vi "Seq AE.vi"(0 "Action":enum16{"READ", "BUILD", "WRITE", "DELETE"}(ring), 3 "Cluster":T5 {"Laser Parameters Out"."STED Power (V)" scale=0.0..10.0; "Image Acquisition Parameters Out"."Z Steps Size (um)" min=0.0; "Image Acquisition Parameters Out"."Number of Z Steps" min=1; "Image Acquisition Parameters Out"."Frames Accumulations" min=1; "Image Acquisition Parameters Out"."Frames Per Capture" min=1; "Image Acquisition Parameters Out"."Line Accumulations" min=1; "Image Acquisition Parameters Out"."Image Format" items=["64 x 64"=64, "128 x 128"=128, "256 x 256"=256, "512 x 512"=512, "1024 x 1024"=1024, "2048 x 2048"=2048, "Customized..."=0]}) -> (9 "Array":T4(array[cluster]) {"Laser Parameters Out"."STED Power (V)" scale=0.0..10.0; "Image Acquisition Parameters Out"."Z Steps Size (um)" min=0.0; "Image Acquisition Parameters Out"."Number of Z Steps" min=1; "Image Acquisition Parameters Out"."Frames Accumulations" min=1; "Image Acquisition Parameters Out"."Frames Per Capture" min=1; "Image Acquisition Parameters Out"."Line Accumulations" min=1; "Image Acquisition Parameters Out"."Image Format" items=["64 x 64"=64, "128 x 128"=128, "256 x 256"=256, "512 x 512"=512, "1024 x 1024"=1024, "2048 x 2048"=2048, "Customized..."=0]})   [LabVIEW 2014]
uses:
  Detectors.ctl
  Laser Controls.ctl
  Type Defs/Image Acquisition Parameters.ctl
panel:
  # "Length"
  # "Height"
  # "XY"
  # "Z"
  # "Length"
  # "Height"
  # "Length"
  # "Height"
  # "XY"
  # "Z"
  # "Length"
  # "Height"
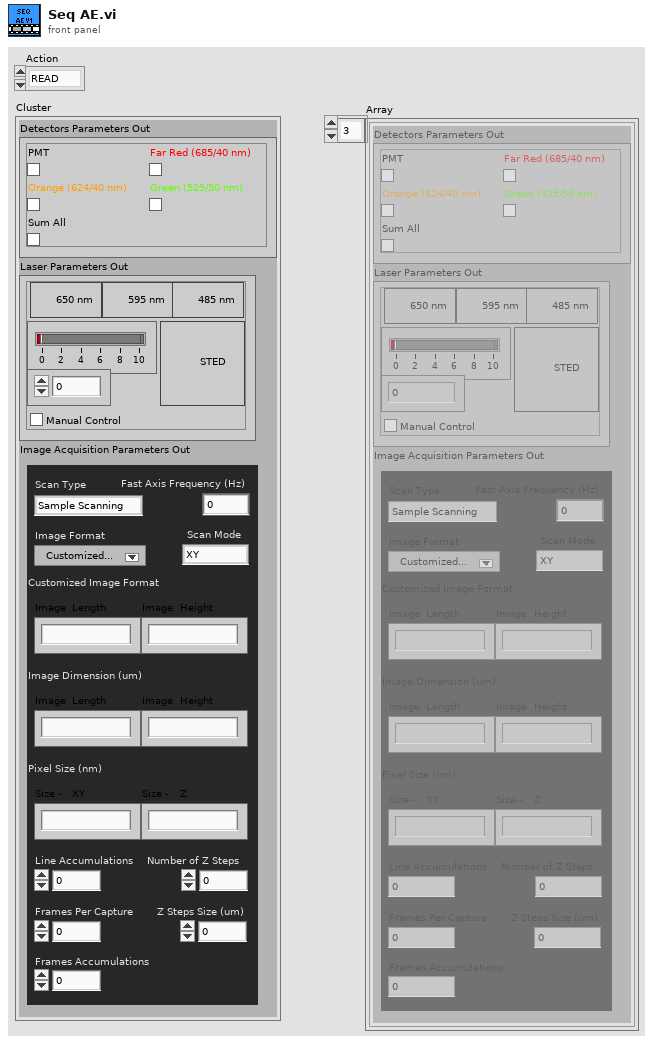
[diagram p1: front panel]
types:
  T1 = typedef "Detectors.ctl" = cluster{"PMT":bool, "Far Red (685/40 nm)":bool, "Orange (624/40 nm)":bool, "Green (525/50 nm)":bool, "Sum All":bool}
  T2 = typedef "Laser Controls.ctl" = cluster{"STED Power (V)":dbl, "STED":bool, "650 nm":bool, "590 nm":bool, "485 nm":bool, "Manual Control":bool}
  T3 = typedef "Image Acquisition Parameters.ctl" = cluster{"Scan Type":enum16{"Sample Scanning", "Beam Scanning"}, "Scan Mode":enum16{"XY", "XZ", "YZ", "XYZ"}, "Fast Axis Frequency (Hz)":dbl, "Image Format":u16, "Line Accumulations":u16, "Frames Per Capture":u16, "Frames Accumulations":u16, "Image Dimension (um)":dbl[], "Number of Z Steps":u16, "Z Steps Size (um)":dbl, "Pixel Size (nm)":dbl[], "Customized Image Format":dbl[]}
  T4 = cluster{"Detectors Parameters Out":T1, "Laser Parameters Out":T2, "Image Acquisition Parameters Out":T3}[]
  T5 = cluster{"Detectors Parameters Out":T1, "Laser Parameters Out":T2, "Image Acquisition Parameters Out":T3}
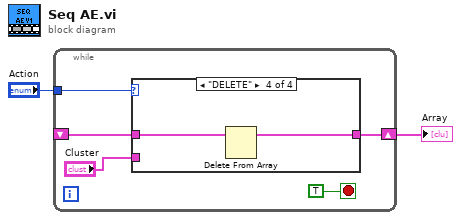
[diagram p0: block diagram]
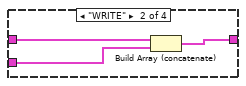
[diagram p3: hidden frame]
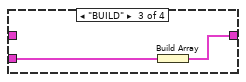
[diagram p4: hidden frame]
diagram:
  n1 = while {
    tunnel: "Action" -> [w6]
    shift-right: [w5] -> w1
    shift-left: _ -> [w4]
    stop <- TRUE stop-if-true
    n2 = case shown="\"DELETE\"" w6 {
      tunnel: [w8 w9 w13 w14] -> w5
      tunnel: w4 -> [w8 w11 _ w15]
      tunnel: "Cluster" -> [_ w10 w12 _]
      frame "READ", Default {
      }
      frame "WRITE" {
        n3 = Build Array (concatenate)(w11, w10) -> (w9:T4)
      }
      frame "BUILD" {
        n4 = Build Array(w12) -> (w13:T4)
      }
      frame "DELETE" {
        n5 = Delete From Array(array=w15) -> (array with subset deleted=w14:T4)  [unwired: 2 in, 1 out]
      }
    }
  }
  "Array" <- w1
